vi "GUI.Config Test BORRAR.vi"() -> ()   [LabVIEW 2009]
uses:
  Test.ctl
  TEST.TEST CONFIG HW.ctl
  Rigol DP832/DP832_Control Channels.ctl
  TEST.TEST CONFIG TEST MATRIZ.ctl
  TEST.TEST CONFIG TEST.ctl
  TEST.TEST RESULT.ctl
  test_result fvasic.ctl
  TEST.TEST EXECUTION TEST.ctl
  TEST.TEST CONFIG VGA.ctl
  TEST.TEST TEST INFO.ctl
  TEST.TEST INFO PC.ctl
  machine estate configs.ctl
panel:
  in  "QUIT":bool
  in  "save config":bool
  in  "Load config":bool
  in  "default":bool
  in  "Array":T1(array[cluster]) {"LIMITS OFFSET DIGITAL 3"."MAXIMUM" format="%.3g"; "LIMITS OFFSET ANALOG 2"."MINIMUM" format="%.3g"; "LIMITS OFFSET ANALOG 2"."MAXIMUM" format="%.3g"; "SETUP ADC 2"."MAX DESVIATION ADC" format="%.3g"; "SETUP ADC 2"."NUMBER OF REPETITIONS" format="%.3g"}
  out "xml string":string
  in  "Test":T2={"Config HW"={"VISA Rigol DP832"="Rigol_DP832", "Config Rigol DP832"=[{"Channel"=0, "V Limit"=5.5, "I Limit"=0.5, "V Out"=5.0}, {"Channel"=1, "V Limit"=5.5, "I Limit"=0.8, "V Out"=5.0}, {"Channel"=2, "V Limit"=5.5, "I Limit"=0.2, "V Out"=0.0}], "CTA Test#"="CTA013 A", "FT_Handle"=0, "Espera acceso FT"=10}, "Config Test"=[{"Vasic"=2.8, "Test Register?"=FALSE, "Test ADC?"=FALSE, "Test ADC"={"Repeats ADC"=100, "Max Desviation"=0.1}, "Limits ADC"={"Low"=[1.9, 1.3, 0.65, 0.0, 1.6, 1.4, 1.4, 0.9, 2.1, 0.85, 1.9], "High"=[2.1, 1.5, 0.85, 0.1, 1.4, 1.2, 1.2, 0.7, 1.9, 0.65, 1.7]}, "Test Max PN Min NP?"=FALSE, "Limits Max PN Min NP"={"Max P inferior"=1.888, "Max P superior"=2.177000045776367, "Min N superior"=0.818, "Min N inferior"=0.73, "Max N superior"=1.475, "Max N inferior"=1.322, "Min P inferior "=1.321, "Min P superior"=1.474}, "Test Rate Scan?"=FALSE, "Vin Rate Scan"=[], "Limits Rate Scan"={"High"=[0.15, 0.242, 0.331, 0.425, 0.512, 0.6, 0.688, 0.774, 0.847, 0.91], "Low"=[0.021, 0.11, 0.189, 0.27, 0.347, 0.421, 0.487, 0.551, 0.601, 0.635]}, "Test Rate Scan Adders?"=FALSE, "Vin Rate Adders"=[], "Test offset analog?"=FALSE, "Test offset digital?"=FALSE, "Lim Offset Analog"={"Max Analog"=0.05, "Min Analog"=-0.05}, "Lim offset Dig"={"Max Dig"=0.05}}, {"Vasic"=2.8, "Test Register?"=FALSE, "Test ADC?"=FALSE, "Test ADC"={"Repeats ADC"=100, "Max Desviation"=0.1}, "Limits ADC"={"Low"=[1.9, 1.3, 0.65, 0.0, 1.6, 1.4, 1.4, 0.9, 2.1, 0.85, 1.9], "High"=[2.1, 1.5, 0.85, 0.1, 1.4, 1.2, 1.2, 0.7, 1.9, 0.65, 1.7]}, "Test Max PN Min NP?"=FALSE, "Limits Max PN Min NP"={"Max P inferior"=1.888, "Max P superior"=2.177000045776367, "Min N superior"=0.818, "Min N inferior"=0.73, "Max N superior"=1.475, "Max N inferior"=1.322, "Min P inferior "=1.321, "Min P superior"=1.474}, "Test Rate Scan?"=FALSE, "Vin Rate Scan"=[], "Limits Rate Scan"={"High"=[0.15, 0.242, 0.331, 0.425, 0.512, 0.6, 0.688, 0.774, 0.847, 0.91], "Low"=[0.021, 0.11, 0.189, 0.27, 0.347, 0.421, 0.487, 0.551, 0.601, 0.635]}, "Test Rate Scan Adders?"=FALSE, "Vin Rate Adders"=[], "Test offset analog?"=FALSE, "Test offset digital?"=FALSE, "Lim Offset Analog"={"Max Analog"=0.05, "Min Analog"=-0.05}, "Lim offset Dig"={"Max Dig"=0.05}}, {"Vasic"=2.8, "Test Register?"=FALSE, "Test ADC?"=FALSE, "Test ADC"={"Repeats ADC"=100, "Max Desviation"=0.1}, "Limits ADC"={"Low"=[1.9, 1.3, 0.65, 0.0, 1.6, 1.4, 1.4, 0.9, 2.1, 0.85, 1.9], "High"=[2.1, 1.5, 0.85, 0.1, 1.4, 1.2, 1.2, 0.7, 1.9, 0.65, 1.7]}, "Test Max PN Min NP?"=FALSE, "Limits Max PN Min NP"={"Max P inferior"=1.888, "Max P superior"=2.177000045776367, "Min N superior"=0.818, "Min N inferior"=0.73, "Max N superior"=1.475, "Max N inferior"=1.322, "Min P inferior "=1.321, "Min P superior"=1.474}, "Test Rate Scan?"=FALSE, "Vin Rate Scan"=[], "Limits Rate Scan"={"High"=[0.15, 0.242, 0.331, 0.425, 0.512, 0.6, 0.688, 0.774, 0.847, 0.91], "Low"=[0.021, 0.11, 0.189, 0.27, 0.347, 0.421, 0.487, 0.551, 0.601, 0.635]}, "Test Rate Scan Adders?"=FALSE, "Vin Rate Adders"=[], "Test offset analog?"=FALSE, "Test offset digital?"=FALSE, "Lim Offset Analog"={"Max Analog"=0.05, "Min Analog"=-0.05}, "Lim offset Dig"={"Max Dig"=0.05}}, {"Vasic"=2.8, "Test Register?"=FALSE, "Test ADC?"=FALSE, "Test ADC"={"Repeats ADC"=100, "Max Desviation"=0.1}, "Limits ADC"={"Low"=[1.9, 1.3, 0.65, 0.0, 1.6, 1.4, 1.4, 0.9, 2.1, 0.85, 1.9], "High"=[2.1, 1.5, 0.85, 0.1, 1.4, 1.2, 1.2, 0.7, 1.9, 0.65, 1.7]}, "Test Max PN Min NP?"=FALSE, "Limits Max PN Min NP"={"Max P inferior"=1.888, "Max P superior"=2.177000045776367, "Min N superior"=0.818, "Min N inferior"=0.73, "Max N superior"=1.475, "Max N inferior"=1.322, "Min P inferior "=1.321, "Min P superior"=1.474}, "Test Rate Scan?"=FALSE, "Vin Rate Scan"=[], "Limits Rate Scan"={"High"=[0.15, 0.242, 0.331, 0.425, 0.512, 0.6, 0.688, 0.774, 0.847, 0.91], "Low"=[0.021, 0.11, 0.189, 0.27, 0.347, 0.421, 0.487, 0.551, 0.601, 0.635]}, "Test Rate Scan Adders?"=FALSE, "Vin Rate Adders"=[], "Test offset analog?"=FALSE, "Test offset digital?"=FALSE, "Lim Offset Analog"={"Max Analog"=0.05, "Min Analog"=-0.05}, "Lim offset Dig"={"Max Dig"=0.05}}], "Result"=[], "Execucion Test"={"Vasic Actual"=0}, "Config VGA"={"Theoretical Voltage"=[0.1, 0.2, 0.3, 0.4, 0.5, 0.6, 0.7, 0.8, 0.9, 1.0], "Real Voltage"=[0.10285, 0.20714, 0.29957, 0.40485, 0.49571, 0.60685, 0.69771, 0.80114, 0.89714, 0.99885], "Pulse Width"=57344, "Frecuency Pulse"=1000000.0, "VGA Gain"=[9, 16, 24, 34, 43, 52, 61, 72, 81, 93]}, "Test Info"={"Asic"="", "Operator"="", "Place"="", "Time start"=timestamp(0 s since 1904-01-01), "Time stop"=timestamp(0 s since 1904-01-01)}, "Info machine"={"SO"="", "SO Name"="", "SO Ver"="", "SO Build"="", "CPU"="", "APP"="", "APP YEAR"="", "APP ver"="", "APP User"="", "APP Serail"="", "MAC"=[], "PC NAME"=[], "PC IP"=[], "BIOS MANU"="", "BIOS NAME"="", "BIOS SERIAL"="", "BOARD MANU"="", "BOARD NAME"="", "BOARD SERIAL"="", "Driver Version"="", "Library Version"=""}} {"Config VGA"."Theoretical Voltage" format="%1.4f"; "Config VGA"."VGA Gain" format="%02x"; "Config VGA"."Frecuency Pulse" format="%0_2p"; "Config VGA"."Pulse Width" format="%04x"; "Config VGA"."Real Voltage" format="%1.5f"; "Config Test"."Limits ADC"."High" format="%1.4f"; "Config Test"."Limits ADC"."Low" format="%1.3f"; "Config Test"."Lim offset Dig"."Max Dig" format="%.3g"; "Config Test"."Lim Offset Analog"."Min Analog" format="%.3g"; "Config Test"."Lim Offset Analog"."Max Analog" format="%.3g"; "Config Test"."Limits Rate Scan"."Low" format="%1.4f"; "Config Test"."Limits Rate Scan"."High" format="%1.3f"; "Config Test"."Limits Max PN Min NP"."Min P superior" format="%.3g"; "Config Test"."Limits Max PN Min NP"."Min P inferior" format="%.3g"; "Config Test"."Limits Max PN Min NP"."Max N inferior" format="%.3g"; "Config Test"."Limits Max PN Min NP"."Max N superior" format="%.3g"; "Config Test"."Limits Max PN Min NP"."Min N inferior" format="%.3g"; "Config Test"."Limits Max PN Min NP"."Min N superior" format="%.3g"; "Config Test"."Limits Max PN Min NP"."Max P superior" format="%.3g"; "Config Test"."Limits Max PN Min NP"."Max P inferior" format="%.3g"; "Config Test"."Vasic" min=2.8 max=3.8 step=0.01 format="%.2g"; "Config HW"."Config Rigol DP832"."Channel" items=["+30V Channel 1", "+30V Channel 2", "+5V Channel 3"]; "Config HW"."Config Rigol DP832"."V Limit" format="%.1g"; "Config HW"."Config Rigol DP832"."I Limit" format="%.1g"; "Config HW"."Config Rigol DP832"."V Out" format="%.1g"; "Result"."Test Registros"."Read W/R" format="%04x"; "Result"."Test Registros"."Pattern W/R" format="%04x"; "Result"."Test Registros"."Read Default" format="%04x"; "Result"."Test Registros"."Pattern Default" format="%04x"}
  in  "visualize":enum32{"Page 1", "Page 2"}(tab)
  in  "CONFIGURACION PRUEBA":T13(tab)
  in  "Ruta Destino":path
  in  "Place":string(combo)
  in  "Operator's Name":string(combo)
  out "ASIC'S Number":string
  in  "CONFIG TESTS":T14(tab)
  in  "SETUP ADC":T15={"NUMBER OF REPETITIONS"=0.05, "MAX DESVIATION ADC"=-0.05} {"MAX DESVIATION ADC" format="%.3g"; "NUMBER OF REPETITIONS" format="%.3g"}
  in  "LIMITS MEASUREMENT ADC":string[][](table)
  in  "TEST ADC":bool
  in  "LIMITS MAX PN MIN NP":string[][](table)
  in  "TEST MAX MIN P/N":bool
  in  "VIN ASIC":i32[](listbox)
  in  "LIMITS RATE SCAN":string[][](table)
  in  "TEST RATE SCAN":bool
  in  "VIN ASIC ADD":i32[](listbox)
  in  "LIMITS RATE SCAN ADDERS":string[][](table)
  in  "TEST RATE SCAN ADDERS":bool
  in  "LIMITS OFFSET ANALOG":cluster{"MAXIMUM":dbl, "MINIMUM":dbl}={"MAXIMUM"=0.05, "MINIMUM"=-0.05} {"MINIMUM" format="%.3g"; "MAXIMUM" format="%.3g"}
  in  "TEST OFFSET ANALOG":bool
  in  "LIMITS OFFSET DIGITAL":cluster{"MAXIMUM":dbl}={"MAXIMUM"=0.05} {"MAXIMUM" format="%.3g"}
  in  "TEST OFFSET DIGITAL":bool
  in  "VSUPPLY ASIC":string[][](table)
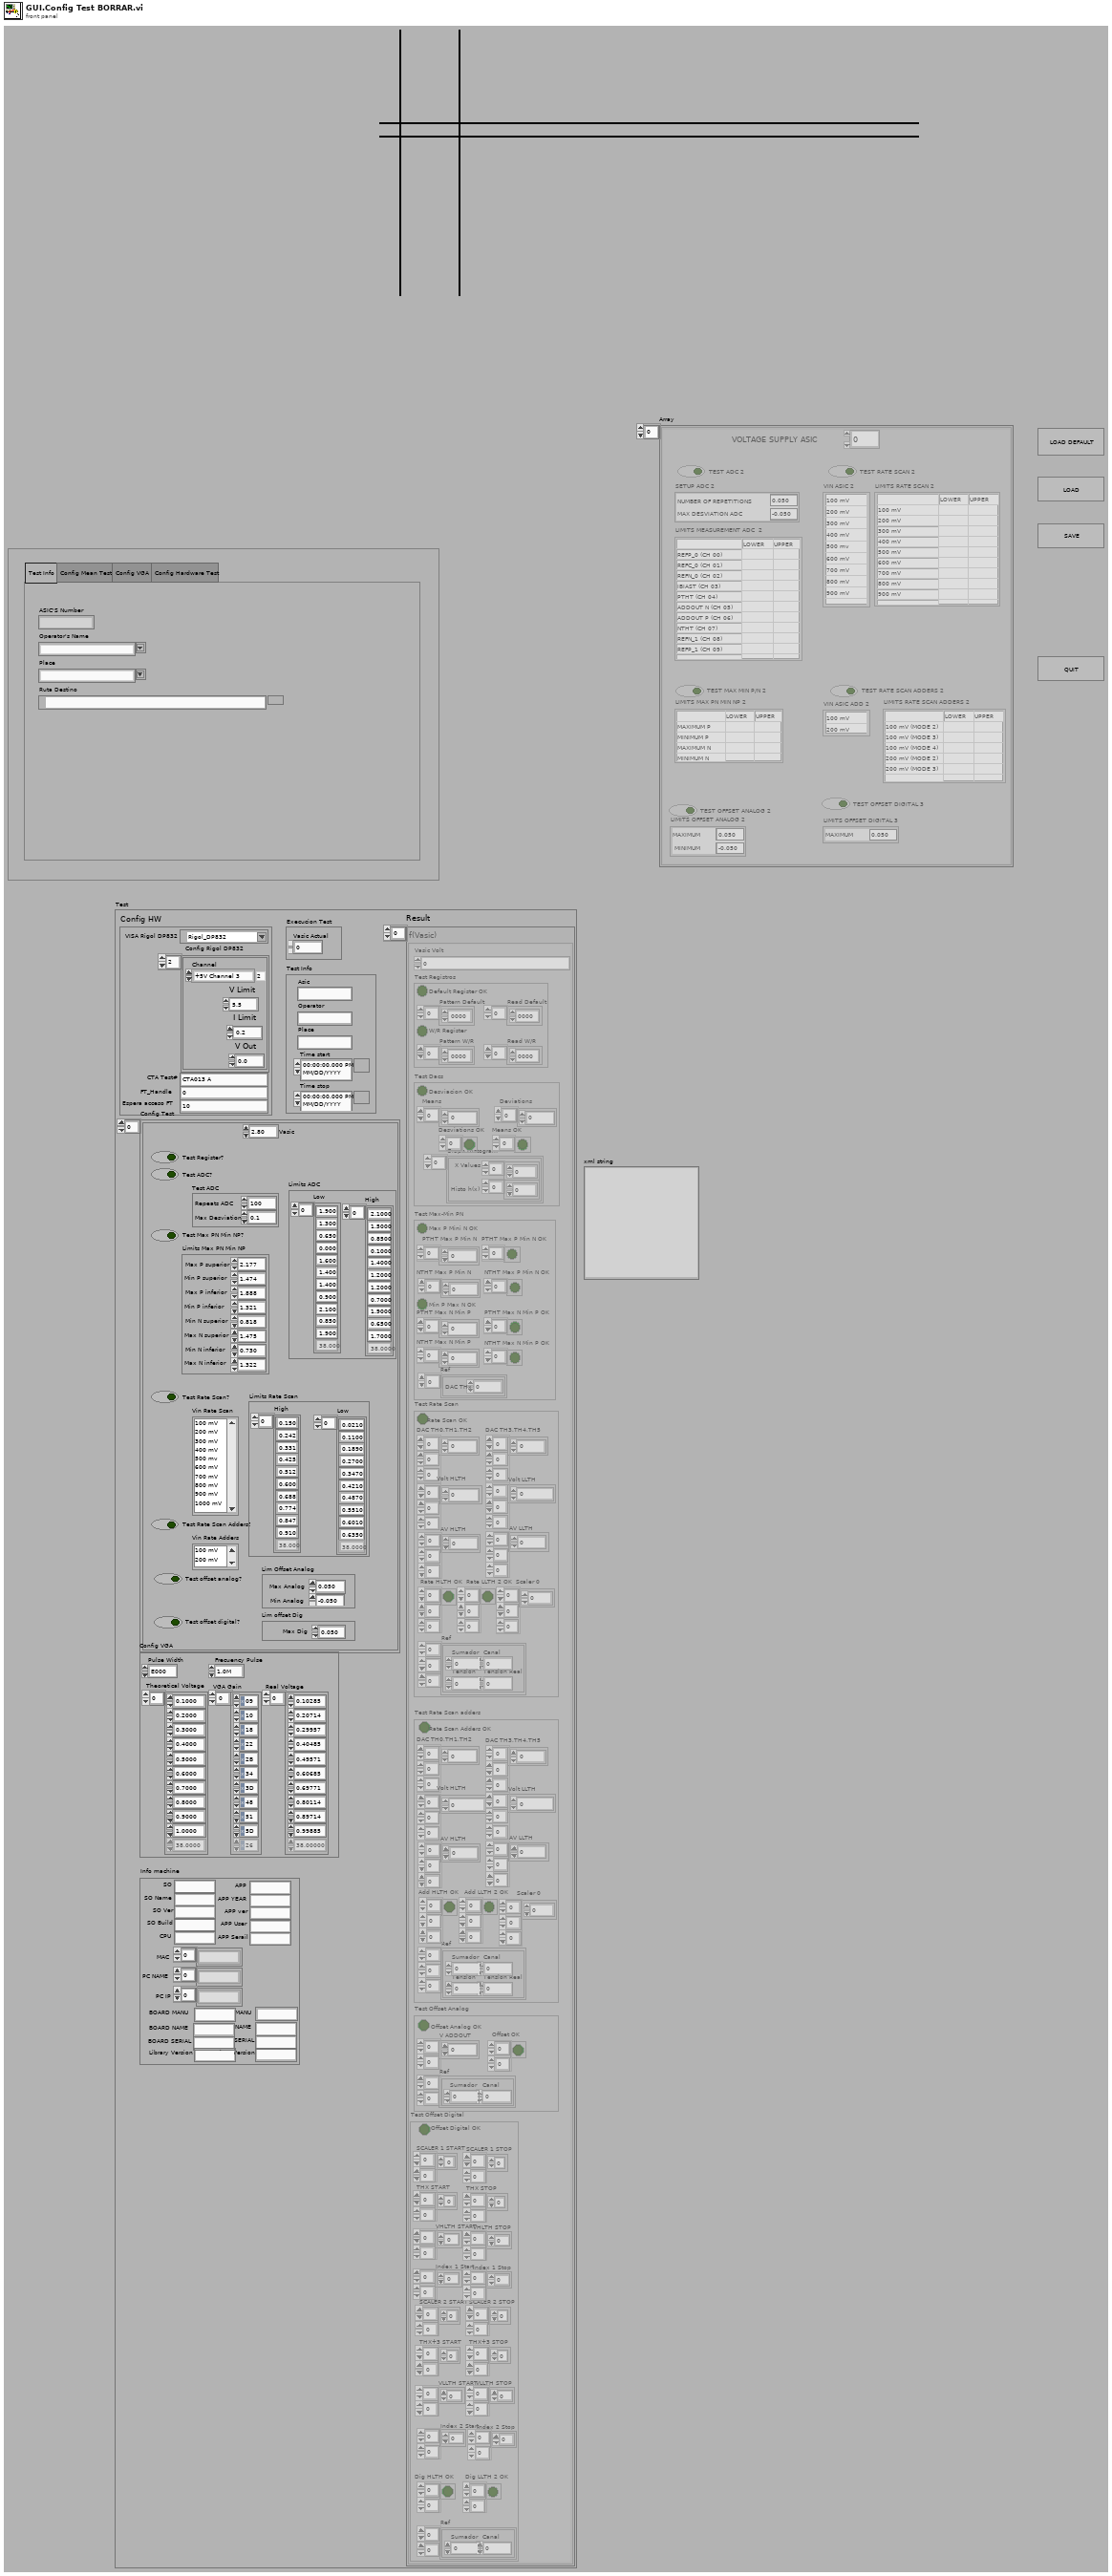
[diagram p1: front panel]
types:
  T1 = cluster{"TEST ADC 2":bool, "SETUP ADC 2":cluster{"NUMBER OF REPETITIONS":dbl, "MAX DESVIATION ADC":dbl}, "LIMITS MEASUREMENT ADC  2":string[][], "TEST MAX MIN P/N 2":bool, "LIMITS MAX PN MIN NP 2":string[][], "TEST RATE SCAN 2":bool, "VIN ASIC 2":i32[], "LIMITS RATE SCAN 2":string[][], "TEST RATE SCAN ADDERS 2":bool, "VIN ASIC ADD 2":i32[], "LIMITS RATE SCAN ADDERS 2":string[][], "TEST OFFSET ANALOG 2":bool, "LIMITS OFFSET ANALOG 2":cluster{"MAXIMUM":dbl, "MINIMUM":dbl}, "TEST OFFSET DIGITAL 3":bool, "LIMITS OFFSET DIGITAL 3":cluster{"MAXIMUM":dbl}, "VOLTAGE SUPPLY ASIC":dbl}[]
  T2 = typedef "Test.ctl" = cluster{"Config HW":T3, "Config Test":T5, "Result":T7, "Execucion Test":T9, "Config VGA":T10, "Test Info":T11, "Info machine":T12}
  T3 = typedef "TEST.TEST CONFIG HW.ctl" = cluster{"VISA Rigol DP832":refnum<visa-resource-name>, "Config Rigol DP832":cluster{"Channel":T4, "V Limit":dbl, "I Limit":dbl, "V Out":dbl}[], "CTA Test#":string, "FT_Handle":u32, "Espera acceso FT":u32}
  T4 = typedef "DP832_Control Channels.ctl" = i32
  T5 = typedef "TEST.TEST CONFIG TEST MATRIZ.ctl" = T6[]
  T6 = typedef "TEST.TEST CONFIG TEST.ctl" = cluster{"Vasic":dbl, "Test Register?":bool, "Test ADC?":bool, "Test ADC":cluster{"Repeats ADC":i32, "Max Desviation":dbl}, "Limits ADC":cluster{"Low":dbl[], "High":dbl[]}, "Test Max PN Min NP?":bool, "Limits Max PN Min NP":cluster{"Max P inferior":dbl, "Max P superior":dbl, "Min N superior":dbl, "Min N inferior":dbl, "Max N superior":dbl, "Max N inferior":dbl, "Min P inferior ":dbl, "Min P superior":dbl}, "Test Rate Scan?":bool, "Vin Rate Scan":i32[], "Limits Rate Scan":cluster{"High":dbl[], "Low":dbl[]}, "Test Rate Scan Adders?":bool, "Vin Rate Adders":i32[], "Test offset analog?":bool, "Test offset digital?":bool, "Lim Offset Analog":cluster{"Max Analog":dbl, "Min Analog":dbl}, "Lim offset Dig":cluster{"Max Dig":dbl}}
  T7 = typedef "TEST.TEST RESULT.ctl" = T8[]
  T8 = typedef "test_result fvasic.ctl" = cluster{"Vasic Volt":i32, "Test Registros":cluster{"Default Register OK":bool, "Pattern Default":u16[], "Read Default":u16[], "W/R Register":bool, "Pattern W/R":u16[], "Read W/R":u16[]}, "Test Dacs":cluster{"Desviacion OK":bool, "Means":dbl[], "Deviations":dbl[], "Desviations OK":bool[], "Means OK":bool[], "Graph Histogram":cluster{"X Values":dbl[], "Histo h(x)":i32[]}[]}, "Test Max-Min PN":cluster{"Max P Mini N OK":bool, "PTHT Max P Min N":dbl[], "PTHT Max P Min N OK":bool[], "NTHT Max P Min N":dbl[], "NTHT Max P Min N OK":bool[], "Min P Max N OK":bool, "PTHT Max N Min P":dbl[], "PTHT Max N Min P OK":bool[], "NTHT Max N Min P":dbl[], "NTHT Max N Min P OK":bool[], "Ref":cluster{"DAC THx":u8}[]}, "Test Rate Scan":cluster{"Rate Scan OK":bool, "DAC TH0,TH1,TH2":u16[][][], "Volt HLTH":dbl[][][], "AV HLTH":dbl[][][], "Rate HLTH OK":bool[][][], "DAC TH3,TH4,TH5":u16[][][], "Volt LLTH":dbl[][][], "AV LLTH":dbl[][][], "Rate LLTH 2 OK":bool[][][], "Scaler 0":u16[][][], "Ref":cluster{"Sumador":u8, "Canal":u8, "Tension":u8, "Tension Real":dbl}[][][]}, "Test Rate Scan adders":cluster{"Rate Scan Adders OK":bool, "DAC TH0,TH1,TH2":u16[][][], "Volt HLTH":dbl[][][], "AV HLTH":dbl[][][], "Add HLTH OK":bool[][][], "DAC TH3,TH4,TH5":u16[][][], "Volt LLTH":dbl[][][], "AV LLTH":dbl[][][], "Add LLTH 2 OK":bool[][][], "Scaler 0":u16[][][], "Ref":cluster{"Sumador":u8, "Canal":u8, "Tension":u8, "Tension Real":dbl}[][][]}, "Test Offset Analog":cluster{"Offset Analog OK":bool, "V ADDOUT":dbl[][], "Offset OK":bool[][], "Ref":cluster{"Sumador":u8, "Canal":u8}[][]}, "Test Offset Digital":cluster{"Offset Digital OK":bool, "SCALER 1 START":u16[][], "SCALER 1 STOP":u16[][], "THX START":u16[][], "THX STOP":u16[][], "VHLTH START":dbl[][], "VHLTH STOP":dbl[][], "Index 1 Start":i32[][], "index 1 Stop":i32[][], "SCALER 2 START":u16[][], "SCALER 2 STOP":u16[][], "THX+3 START":u16[][], "THX+3 STOP":u16[][], "VLLTH START":dbl[][], "VLLTH STOP":dbl[][], "Index 2 Start":i32[][], "index 2 Stop":i32[][], "Dig HLTH OK":bool[][], "Dig LLTH 2 OK":bool[][], "Ref":cluster{"Sumador":u8, "Canal":u8}[][]}}
  T9 = typedef "TEST.TEST EXECUTION TEST.ctl" = cluster{"Vasic Actual":i32}
  T10 = typedef "TEST.TEST CONFIG VGA.ctl" = cluster{"Theoretical Voltage":dbl[], "Real Voltage":dbl[], "Pulse Width":u16, "Frecuency Pulse":dbl, "VGA Gain":u8[]}
  T11 = typedef "TEST.TEST TEST INFO.ctl" = cluster{"Asic":string, "Operator":string, "Place":string, "Time start":timestamp, "Time stop":timestamp}
  T12 = typedef "TEST.TEST INFO PC.ctl" = cluster{"SO":string, "SO Name":string, "SO Ver":string, "SO Build":string, "CPU":string, "APP":string, "APP YEAR":string, "APP ver":string, "APP User":string, "APP Serail":string, "MAC":string[], "PC NAME":string[], "PC IP":string[], "BIOS MANU":string, "BIOS NAME":string, "BIOS SERIAL":string, "BOARD MANU":string, "BOARD NAME":string, "BOARD SERIAL":string, "Driver Version":string, "Library Version":string}
  T13 = enum32{"Test Info", "Config Mean Test", "Config VGA", "Config Hardware Test"}
  T14 = enum32{"ADC", "MAX MIN P/N", "RATE SCAN", "RATE SCAN ADDERS", "OFFSET ANALOG", "OFFSET DIGITAL"}
  T15 = cluster{"NUMBER OF REPETITIONS":dbl, "MAX DESVIATION ADC":dbl}
  T16 = typedef "machine estate configs.ctl" = enum16{"Init", "wait", "Load", "Refresh", "quit", "save", "quit save"}
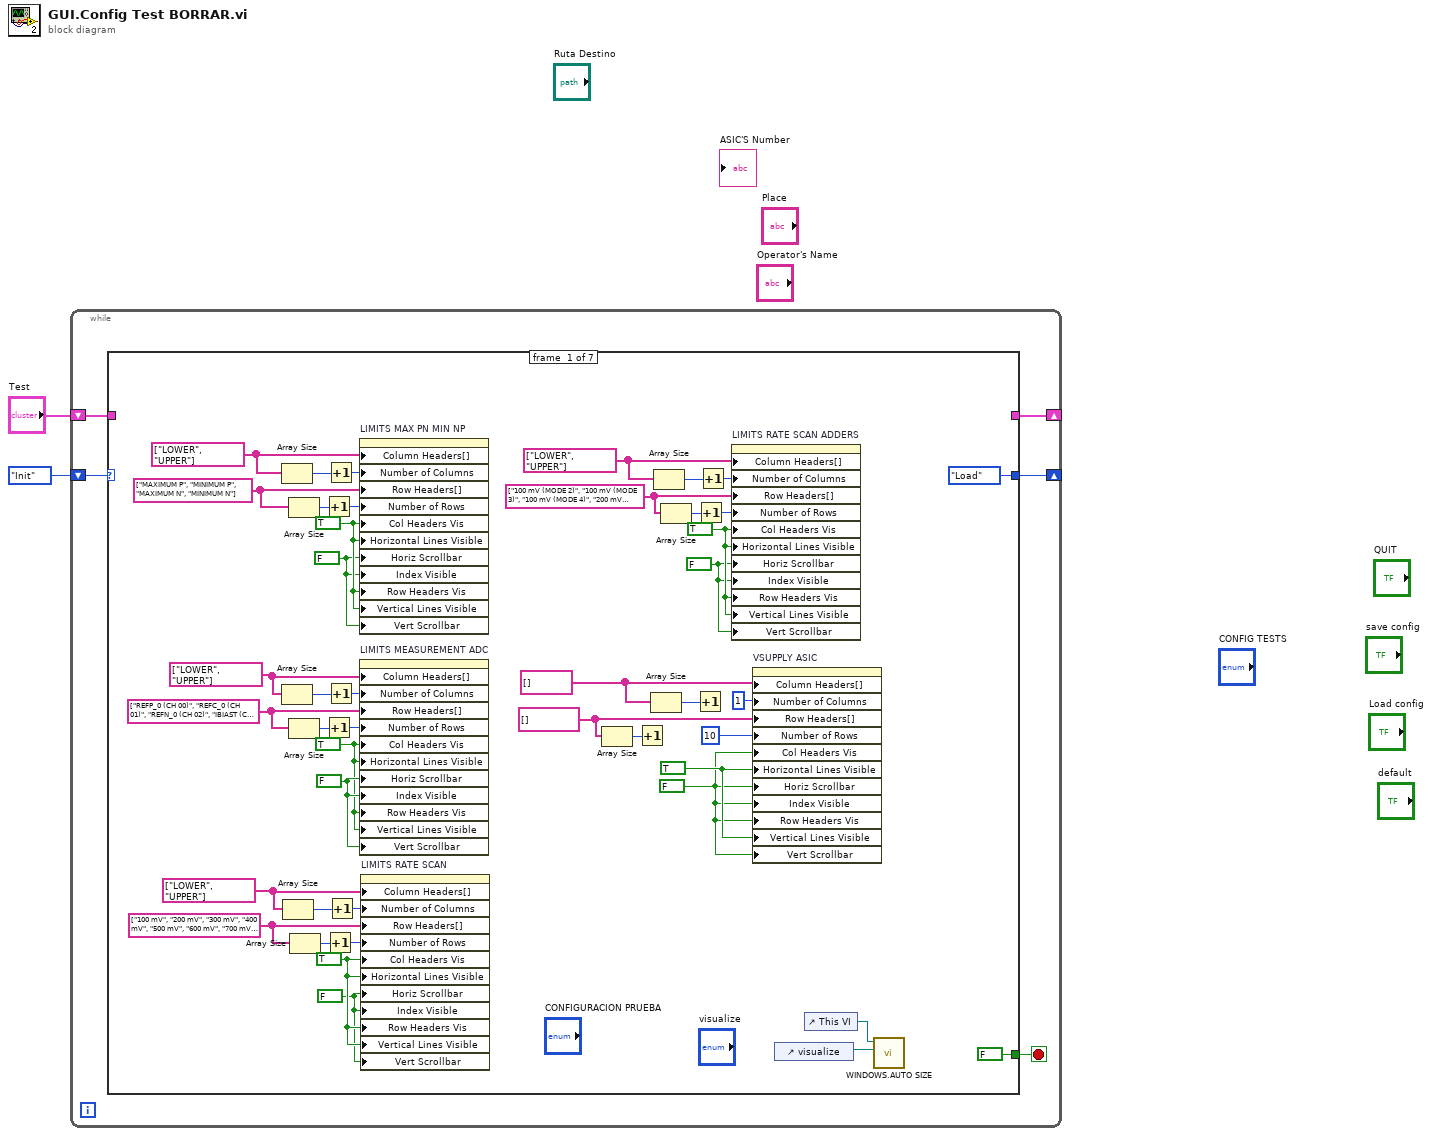
[diagram p0: block diagram]
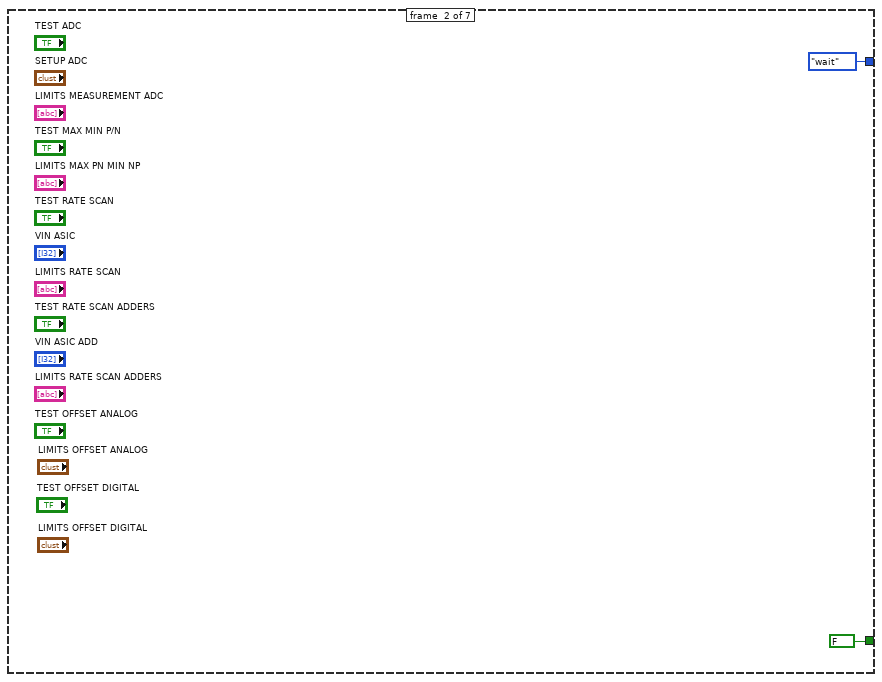
[diagram p2: hidden frame]
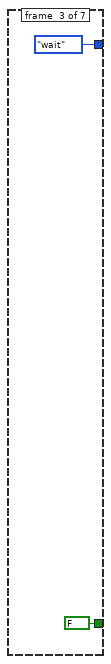
[diagram p3: hidden frame]
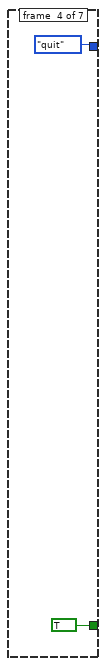
[diagram p4: hidden frame]
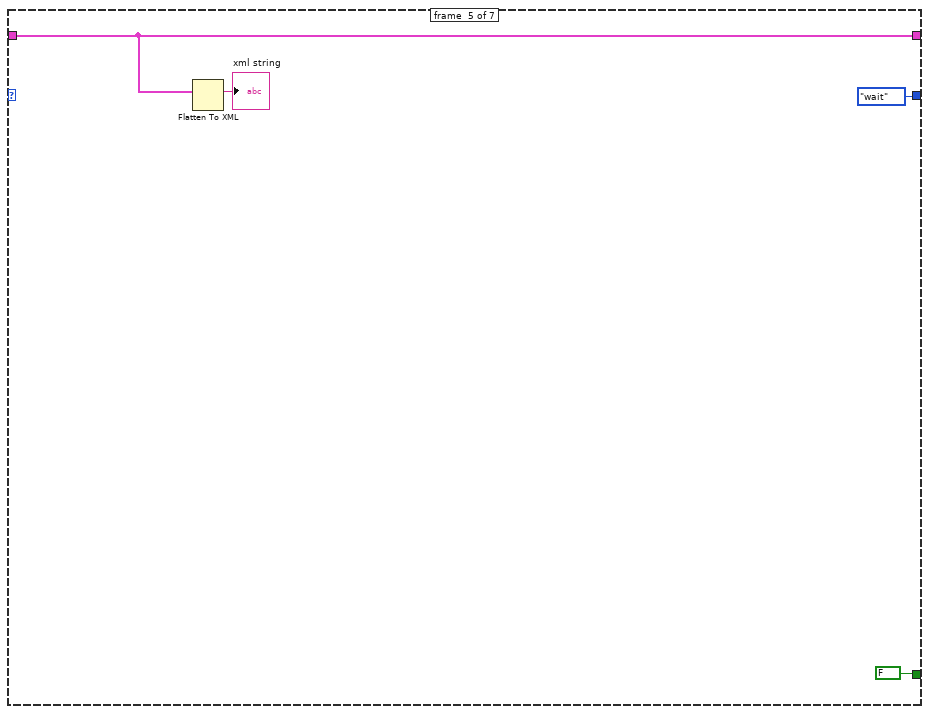
[diagram p5: hidden frame]
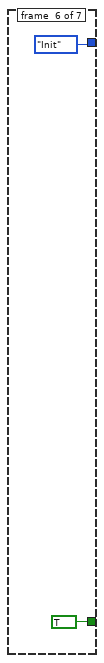
[diagram p6: hidden frame]
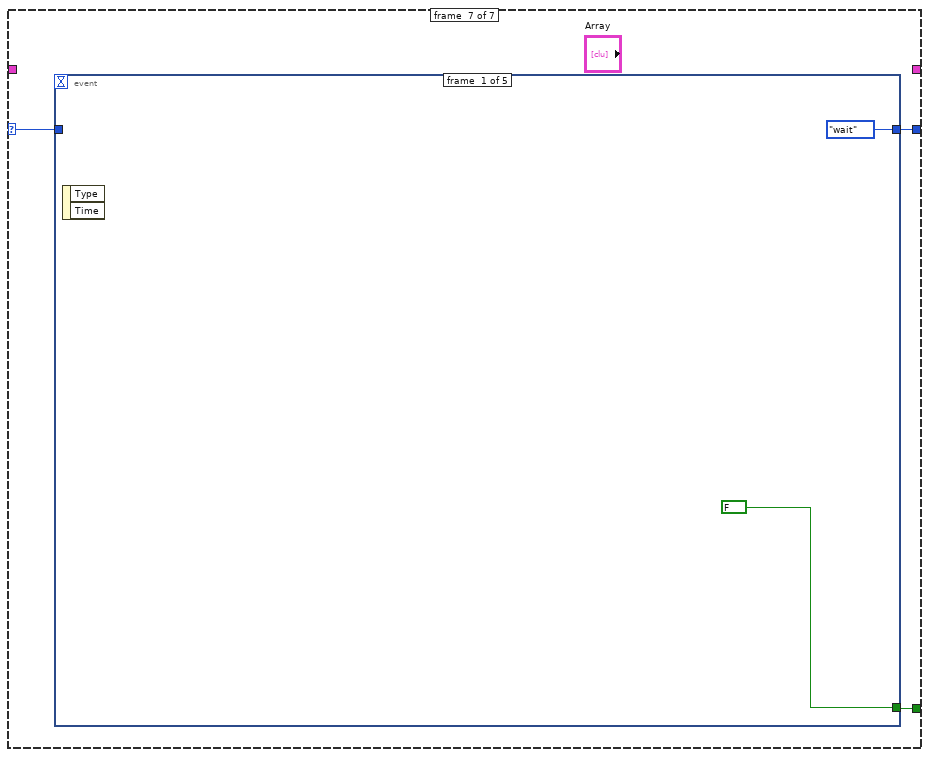
[diagram p7: hidden frame]
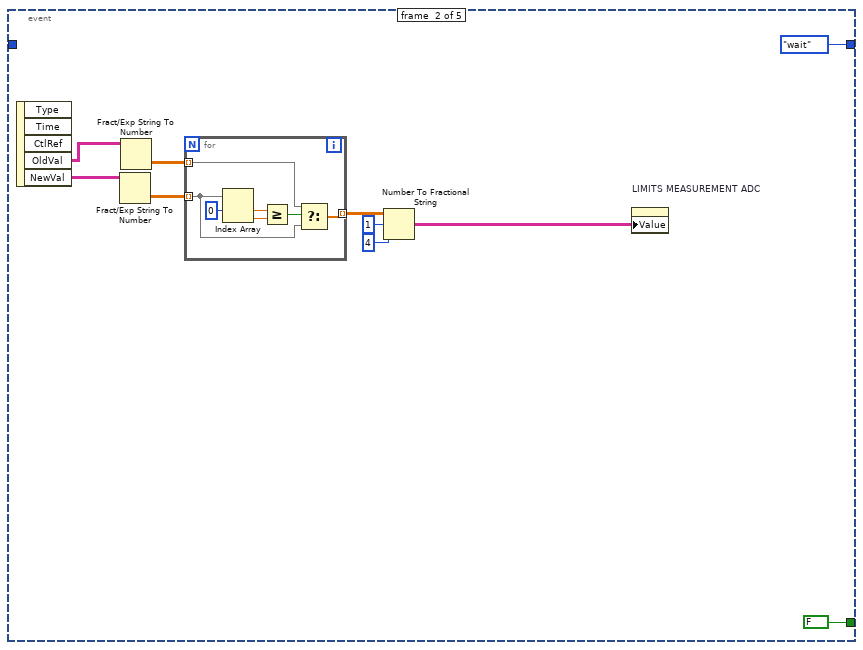
[diagram p8: hidden frame]
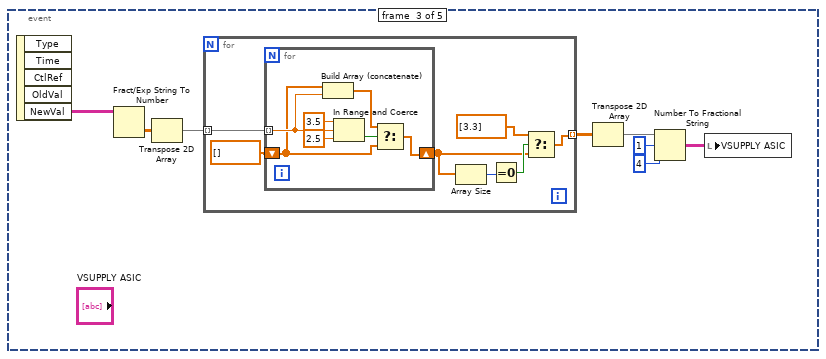
[diagram p9: hidden frame]
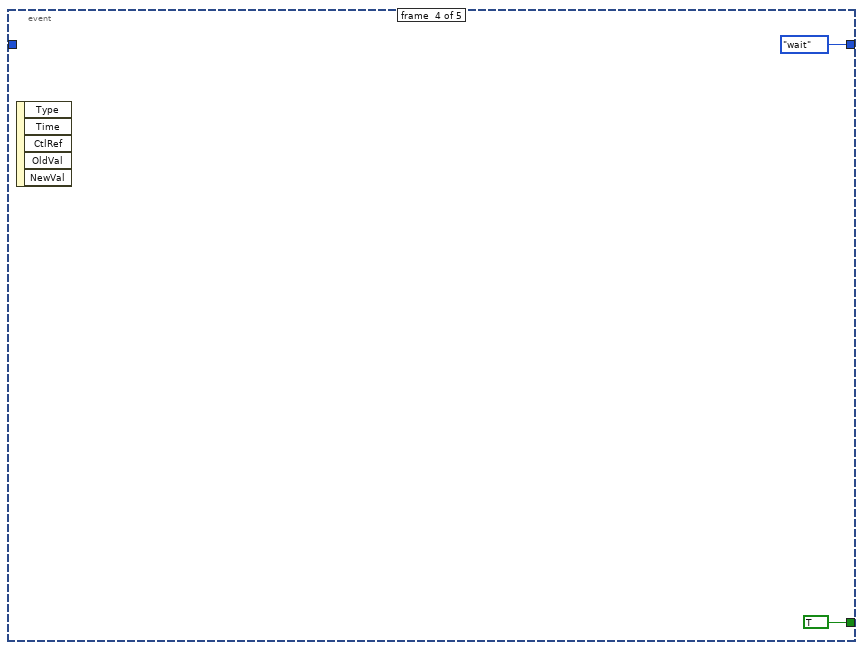
[diagram p10: hidden frame]
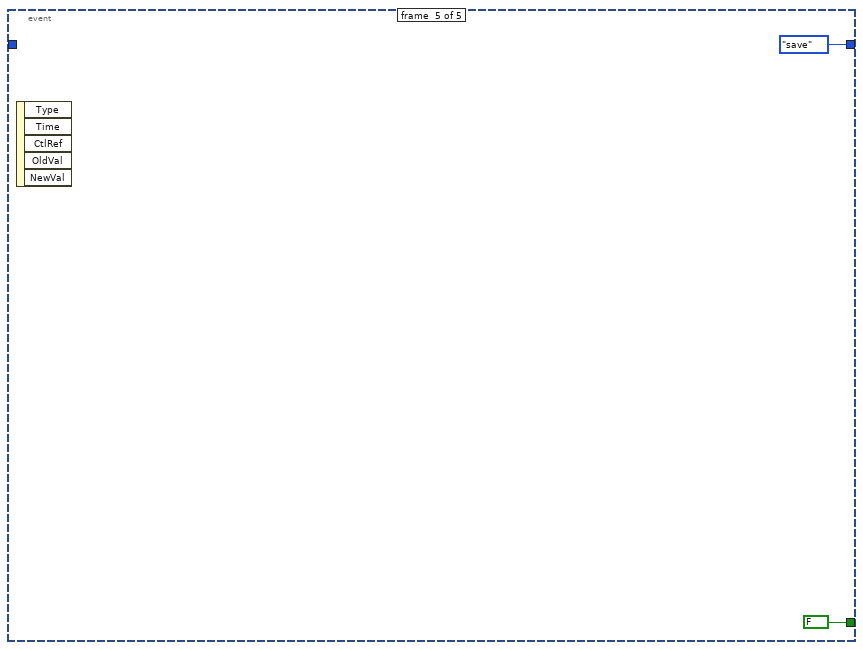
[diagram p11: hidden frame]
diagram:
  n1 = while {
    shift-right: [w5] -> _
    shift-left: machine_estate_configs."Init" ("MACHINE") -> [w6]
    shift-right: [w3] -> _
    shift-left: "Test" -> [w4]
    stop <- w7 stop-if-true
    n2 = case shown="\"wait\"" w6 {
      selector: w6 -> [_ _ _ _ _ _ w65]
      tunnel: [FALSE FALSE FALSE TRUE FALSE TRUE w66] -> w7
      tunnel: [machine_estate_configs."Load" ("MACHINE") machine_estate_configs."wait" ("MACHINE") machine_estate_configs."wait" ("MACHINE") machine_estate_configs."quit" ("MACHINE") machine_estate_configs."wait" ("MACHINE") machine_estate_configs."Init" ("MACHINE") w64] -> w5
      tunnel: w4 -> [_ _ _ _ w58 _ _]
      tunnel: [_ _ _ _ w58 _ _] -> w3
      frame #0 {
        w11 = FALSE ("Autosizing Row Height")
        w12 = TRUE ("Autosizing Row Height")
        w18 = string[] ["LOWER", "UPPER"] ("Column Headers")
        w17 = string[] ["100 mV (MODE 2)", "100 mV (MODE 3)", "100 mV (MODE 4)", "200 mV (MODE 2)", "200 mV (MODE 3)", "200 mV (MODE 2)"] ("Column Headers")
        w8 = FALSE ("Autosizing Row Height")
        w25 = TRUE ("Autosizing Row Height")
        w21 = string[] [] ("Column Headers")
        w22 = string[] [] ("Column Headers")
        w26 = FALSE ("Autosizing Row Height")
        w27 = TRUE ("Autosizing Row Height")
        w33 = string[] ["LOWER", "UPPER"] ("Column Headers")
        w32 = string[] ["100 mV", "200 mV", "300 mV", "400 mV", "500 mV", "600 mV", "700 mV", "800 mV", "900 mV", "1000 mV"] ("Column Headers")
        w34 = FALSE ("Autosizing Row Height")
        w35 = TRUE ("Autosizing Row Height")
        w41 = string[] ["LOWER", "UPPER"] ("Column Headers")
        w40 = string[] ["MAXIMUM P", "MINIMUM P", "MAXIMUM N", "MINIMUM N"] ("Column Headers")
        w51 = FALSE ("Autosizing Row Height")
        w50 = TRUE ("Autosizing Row Height")
        w44 = string[] ["LOWER", "UPPER"] ("Column Headers")
        w45 = string[] ["REFP_0 (CH 00)", "REFC_0 (CH 01)", "REFN_0 (CH 02)", "IBIAST (CH 03)", "PTHT (CH 04)", "ADDOUT N (CH 05)", "ADDOUT P (CH 06)", "NTHT (CH 07)", "REFN_1 (CH 08)", "REFP_1 (CH 09)", "VCOM (CH 10)"] ("Column Headers")
        n3 = Array Size(array=w41) -> (size(s)=w39:i32)
        n4 = Array Size(array=w44) -> (size(s)=w46:i32)
        n5 = Array Size(array=w33) -> (size(s)=w31:i32)
        n6 = Array Size(array=w40) -> (size(s)=w38:i32)
        n7 = Array Size(array=w45) -> (size(s)=w47:i32)
        n8 = Array Size(array=w32) -> (size(s)=w30:i32)
        n9 = Increment(x=w38) -> (x+1=w36:i32)
        n10 = Increment(x=w47) -> (x+1=w49:i32)
        n11 = Increment(x=w30) -> (x+1=w28:i32)
        n12 = Increment(x=w39) -> (x+1=w37:i32)
        n13 = Increment(x=w46) -> (x+1=w48:i32)
        n14 = Increment(x=w31) -> (x+1=w29:i32)
        n15 = property on="LIMITS MAX PN MIN NP" class="Tbl (strict)"("Column Headers[]"=w41, "Number of Columns"=w37, "Row Headers[]"=w40, "Number of Rows"=w36, "Col Headers Vis"=w35, "Horizontal Lines Visible"=w35, "Horiz Scrollbar"=w34, "Index Visible"=w34, "Row Headers Vis"=w35, "Vertical Lines Visible"=w35, "Vert Scrollbar"=w34) -> ()  [unwired: 2 in, 2 out]
        n16 = property on="LIMITS MEASUREMENT ADC" class="Tbl (strict)"("Column Headers[]"=w44, "Number of Columns"=w48, "Row Headers[]"=w45, "Number of Rows"=w49, "Col Headers Vis"=w50, "Horizontal Lines Visible"=w50, "Horiz Scrollbar"=w51, "Index Visible"=w51, "Row Headers Vis"=w50, "Vertical Lines Visible"=w50, "Vert Scrollbar"=w51) -> ()  [unwired: 2 in, 2 out]
        n17 = property on="LIMITS RATE SCAN" class="Tbl (strict)"("Column Headers[]"=w33, "Number of Columns"=w29, "Row Headers[]"=w32, "Number of Rows"=w28, "Col Headers Vis"=w27, "Horizontal Lines Visible"=w27, "Horiz Scrollbar"=w26, "Index Visible"=w26, "Row Headers Vis"=w27, "Vertical Lines Visible"=w27, "Vert Scrollbar"=w26) -> ()  [unwired: 2 in, 2 out]
        n18 = Array Size(array=w22) -> (size(s)=w24:i32)
        n19 = Increment(x=w24) -> ()  [unwired: 1 out]
        n20 = Array Size(array=w21) -> (size(s)=w23:i32)
        n21 = Array Size(array=w18) -> (size(s)=w16:i32)
        n22 = Array Size(array=w17) -> (size(s)=w15:i32)
        n23 = Increment(x=w23) -> ()  [unwired: 1 out]
        n24 = Increment(x=w15) -> (x+1=w13:i32)
        n25 = Increment(x=w16) -> (x+1=w14:i32)
        n26 = property on="LIMITS RATE SCAN ADDERS" class="Tbl (strict)"("Column Headers[]"=w18, "Number of Columns"=w14, "Row Headers[]"=w17, "Number of Rows"=w13, "Col Headers Vis"=w12, "Horizontal Lines Visible"=w12, "Horiz Scrollbar"=w11, "Index Visible"=w11, "Row Headers Vis"=w12, "Vertical Lines Visible"=w12, "Vert Scrollbar"=w11) -> ()  [unwired: 2 in, 2 out]
        n27 = property on="VSUPPLY ASIC" class="Tbl (strict)"("Column Headers[]"=w21, "Number of Columns"=u32 1, "Row Headers[]"=w22, "Number of Rows"=u32 10, "Col Headers Vis"=w8, "Horizontal Lines Visible"=w25, "Horiz Scrollbar"=w8, "Index Visible"=w8, "Row Headers Vis"=w8, "Vertical Lines Visible"=w25, "Vert Scrollbar"=w8) -> ()  [unwired: 2 in, 2 out]
        n28 = control-ref of="visualize"() -> (w19:refnum<vi>)
        n29 = control-ref of="This VI"() -> (w20:refnum<vi>)
        n30 = call "WINDOWS.AUTO SIZE.vi"("TAB.AutoAjuste"=w19, "This VI"=w20) -> ()  [unwired: 5 in, 1 out]
      }
      frame #1 {
      }
      frame #2 {
      }
      frame #3 {
      }
      frame #4 {
        n31 = Flatten To XML(anything=w58) -> (xml string=→"xml string":string)
      }
      frame #5 {
      }
      frame #6 {
        n32 = event shown="[1] \"LIMITS MEASUREMENT ADC \": Value Change" {
          selector: _ -> [_ _ _ _ _]
          dyn-events: _ -> [_ _ _ _ _]
          timeout: _ -> [_ _ _ _ _]
          tunnel: [FALSE FALSE _ TRUE FALSE] -> w66
          tunnel: w65 -> [_ _ _ _ _]
          tunnel: [machine_estate_configs."wait" ("MACHINE") machine_estate_configs."wait" ("MACHINE") _ machine_estate_configs."wait" ("MACHINE") machine_estate_configs."save" ("MACHINE")] -> w64
          event #0 {
            n33 = event-data() -> ()  [unwired: 1 in, 2 out]
          }
          event #1 {
            n34 = event-data() -> ("OldVal"=w72:string[][], "NewVal"=w77:string[][])  [unwired: 1 in, 3 out]
            n35 = Fract/Exp String To Number(string=w77) -> (number=w73:dbl[][])  [unwired: 3 in, 1 out]
            n36 = Fract/Exp String To Number(string=w72) -> (number=w71:dbl[][])  [unwired: 3 in, 1 out]
            n37 = for {
              tunnel: w73 -> [w79] mode=indexing
              tunnel: w71 -> [w80] mode=indexing
              tunnel: [w81] -> w70 mode=indexing
              n38 = Index Array(array=w79, index #1=0 ("index")) -> (element #1=w83:dbl, element #2=w84:dbl)  [unwired: 1 in]
              n39 = Greater Or Equal?(x=w83, y=w84) -> (x >= y?=w82:bool)
              n40 = Select(t=w80, s=w82, f=w79) -> (s? t:f=w81:dbl[])
            }
            n41 = Number To Fractional String(number=w70, width (-)=i16 1, precision (6)=i16 4) -> (F-format string=w78:string[][])  [unwired: 1 in]
            n42 = property on="LIMITS MEASUREMENT ADC" class="Tbl (strict)"("Value"=w78) -> ()  [unwired: 2 in, 2 out]
          }
          event #2 {
            n43 = event-data() -> ("NewVal"=w90:string[][])  [unwired: 1 in, 4 out]
            n44 = Fract/Exp String To Number(string=w90) -> (number=w89:dbl[][])  [unwired: 3 in, 1 out]
            n45 = Transpose 2D Array(2D array=w89) -> (transposed array=w87:dbl[][])
            n46 = for {
              tunnel: w87 -> [w100] mode=indexing
              tunnel: [w94] -> w91 mode=indexing
              n47 = for {
                shift-right: [w101] -> w96
                shift-left: dbl[] [] -> [w102]
                tunnel: w100 -> [w104] mode=indexing
                n48 = Build Array (concatenate)(w102, w104) -> (w103:dbl[])
                n49 = In Range and Coerce(upper limit=3.5, x=w104, lower limit=2.5) -> (In Range?=w105:bool)  [unwired: 1 out]
                n50 = Select(t=w103, s=w105, f=w102) -> (s? t:f=w101:dbl[])
              }
              n51 = Array Size(array=w96) -> (size(s)=w98:i32)
              n52 = Equal To 0?(x=w98) -> (x = 0?=w97:bool)
              n53 = Select(t=dbl[] [3.3], s=w97, f=w96) -> (s? t:f=w94:dbl[])
            }
            n54 = Transpose 2D Array(2D array=w91) -> (transposed array=w86:dbl[][])
            n55 = Number To Fractional String(number=w86, width (-)=i16 1, precision (6)=i16 4) -> (F-format string=w88:string[][])  [unwired: 1 in]
            n56 = local write "VSUPPLY ASIC"(w88) -> ()
          }
          event #3 {
            n57 = event-data() -> ()  [unwired: 1 in, 5 out]
          }
          event #4 {
            n58 = event-data() -> ()  [unwired: 1 in, 5 out]
          }
        }
      }
    }
  }
